vi "Instantiate Py Editor.vi"(11 "error in (no error)":errorcluster) -> (4 "Py Editor in":refnum<class "Py Editor.lvclass">, 15 "error out":errorcluster)   [LabVIEW 2019, in "Py Editor.lvclass"]
uses:
  Py Editor.lvclass
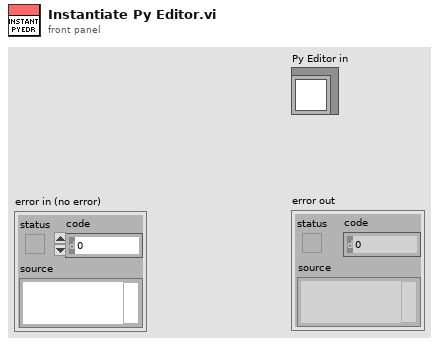
[diagram p1: front panel]
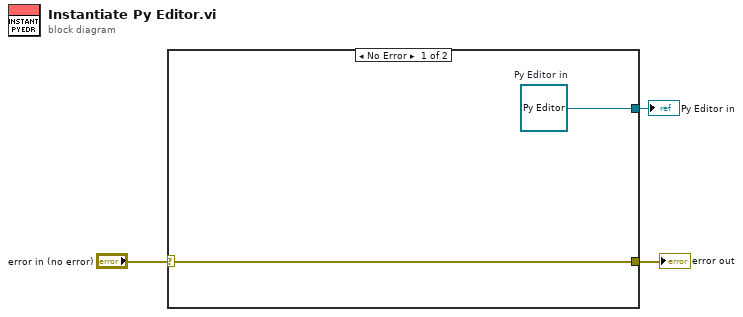
[diagram p0: block diagram]
diagram:
  n1 = case shown="No Error" "error in (no error)" {
    selector: "error in (no error)" -> [w5 w6]
    tunnel: [w5 w6] -> w2
    tunnel: [w4 _] -> w1
    frame No Error {
      w4 = refnum<class "Py Editor.lvclass"> refnum  # Py Editor in
    }
    frame Error {
    }
  }
  "error out" <- w2
  "Py Editor in" <- w1
